vi "Grip System.vi"(10 "Close Grip":bool, 11 "Open Grip":bool) -> ()   [LabVIEW 2018]
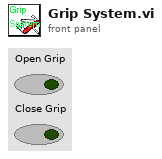
[diagram p1: front panel]
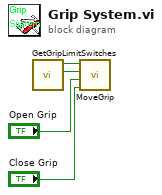
[diagram p0: block diagram]
diagram:
  n1 = call "GetGripLimitSwitches.vi"() -> ("Close Limit Switch"=w3:bool, "Open Limit Switch"=w4:bool)  [unwired: 10 in]
  n2 = call "MoveGrip.vi"("Close Grip"="Close Grip", "Open Grip"="Open Grip", "Close Limit Switch"=w3, "Open Limit Switch"=w4) -> ()  [unwired: 8 in]
